vi "Read Bus Monitor ID.vi"(11 "IBusMonitor":refnum<class "IBusMonitor.lvclass">) -> (3 "Bus Monitor ID":string)   [LabVIEW 2017, in "MonitoredMediator.lvlib" / "IBusMonitor.lvclass"]
uses:
  IBusMonitor.lvclass
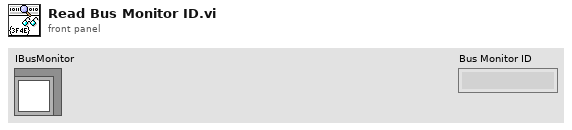
[diagram p1: front panel]
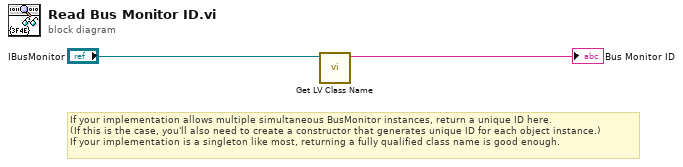
[diagram p0: block diagram]
diagram:
  # "If your implementation allows multiple simultaneous BusMonitor instances, return a unique ID here.\n(If this is the case, you'll also need to create a constructor that generates unique ID for each object instance.)\nIf your implementation is a singleton like most, returning a fully qualified class name is good enough."
  n1 = call <vilib>:"Get LV Class Name.vi"("object"="IBusMonitor") -> ("class name"=→"Bus Monitor ID":string)  [unwired: 9 in, 1 out]
